vi "MTS_Workspace.vi"(6 "Workspace":path, 7 "Operation":T2(ring), 8 "Created in":string, 9 "New Comment":string, 10 "Append File":T1, 11 "Files in Workspace in":T3(array[cluster])) -> (0 "Created":string, 1 "Comment":string, 3 "Files in Workspace":T3(array[cluster]), 4 "Workspace (dup)":path)   [LabVIEW 8.6]
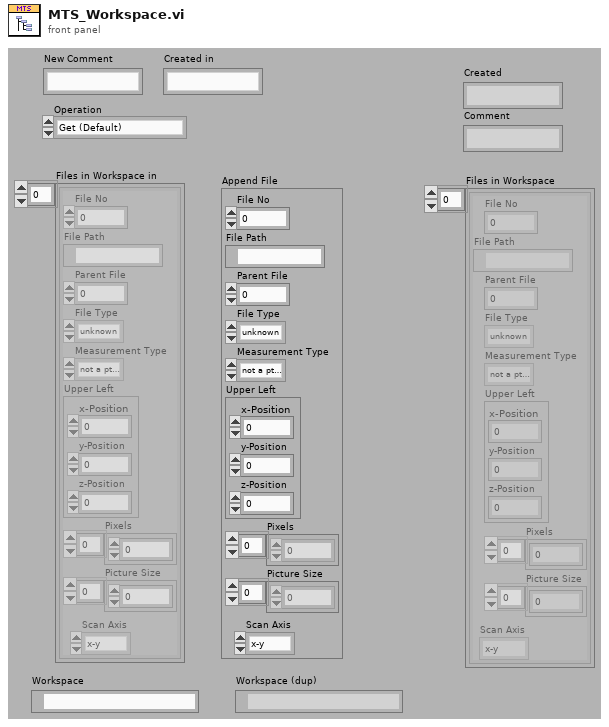
[diagram p1: front panel]
types:
  T1 = cluster{"File No":i32, "File Path":path, "Parent File":i32, "File Type":enum16{"unknown", "pt3 File", "png Image", "bmp Image"}, "Measurement Type":enum16{"not a pt3 File", "Image File", "Point Measurement", "Auto Point"}, "Upper Left":cluster{"x-Position":dbl, "y-Position":dbl, "z-Position":dbl}, "Pixels":i32[], "Picture Size":dbl[], "Scan Axis":enum32{"x-y", "x-z", "y-z"}}
  T2 = enum16{"Get (Default)", "Set Workspace", "Append File", "Change Comment"}
  T3 = cluster{"File No":i32, "File Path":path, "Parent File":i32, "File Type":enum16{"unknown", "pt3 File", "png Image", "bmp Image"}, "Measurement Type":enum16{"not a pt3 File", "Image File", "Point Measurement", "Auto Point"}, "Upper Left":cluster{"x-Position":dbl, "y-Position":dbl, "z-Position":dbl}, "Pixels":i32[], "Picture Size":dbl[], "Scan Axis":enum32{"x-y", "x-z", "y-z"}}[]
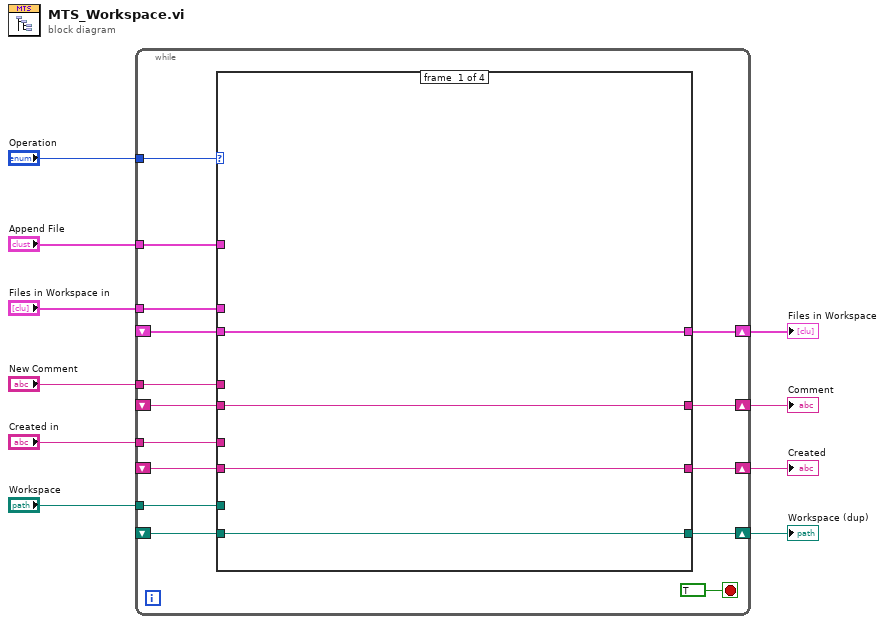
[diagram p0: block diagram]
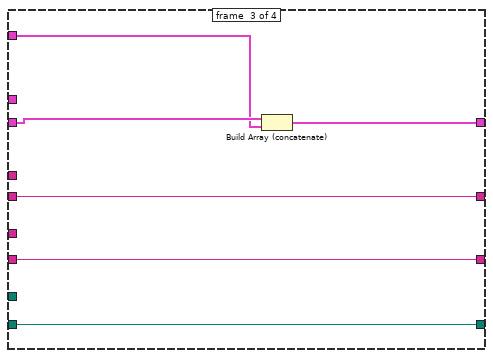
[diagram p3: hidden frame]
diagram:
  n1 = while {
    shift-right: [w24] -> w10
    shift-left: _ -> [w22]
    tunnel: "Operation" -> [w25]
    tunnel: "Files in Workspace in" -> [w23]
    tunnel: "Append File" -> [w21]
    tunnel: "New Comment" -> [w20]
    shift-right: [w19] -> w5
    shift-left: _ -> [w18]
    tunnel: "Created in" -> [w17]
    shift-right: [w16] -> w3
    shift-left: _ -> [w15]
    tunnel: "Workspace" -> [w13]
    shift-right: [w12] -> w1
    shift-left: _ -> [w11]
    stop <- TRUE stop-if-true
    n2 = case shown="\"Change Comment\"" w25 {
      tunnel: [w29 w33 w38 w43] -> w24
      tunnel: w23 -> [_ w33 _ _]
      tunnel: w22 -> [w29 _ w39 w43]
      tunnel: w21 -> [_ _ w37 _]
      tunnel: w20 -> [_ w32 _ w42]
      tunnel: [w28 w32 w36 w42] -> w19
      tunnel: w18 -> [w28 _ w36 _]
      tunnel: w17 -> [_ w31 _ _]
      tunnel: [w27 w31 w35 w41] -> w16
      tunnel: w15 -> [w27 _ w35 w41]
      tunnel: w13 -> [_ w30 _ _]
      tunnel: [w26 w30 w34 w40] -> w12
      tunnel: w11 -> [w26 _ w34 w40]
      frame #0 {
      }
      frame #1 {
      }
      frame #2 {
        n3 = Build Array (concatenate)(w39, w37) -> (w38:T3)
      }
      frame #3 {
      }
    }
  }
  "Files in Workspace" <- w10
  "Created" <- w3
  "Comment" <- w5
  "Workspace (dup)" <- w1
